vi "FPGAmacro6_2.vi"() -> ()   [LabVIEW 2019]
uses:
  <vilib>/Platform/TimedLoop/XDataNode/timing_clust.ctl
  <vilib>/Platform/TimedLoop/XDataNode/nitl_modes.ctl
  <vilib>/Platform/TimedLoop/XDataNode/wakeup.ctl
  <vilib>/rvi/Emulation/niFpgaGetClockAttributes.vi
  <vilib>/rvi/Emulation/niFpgaSctlEmulationGetInTimedLoop.vi
  <vilib>/rvi/Emulation/niFpgaEmulationReportErrorSimple.vi
  <vilib>/rvi/Emulation/niFpgaProcessEmulError.vi
  <vilib>/rvi/eio/common/nirviEmuTemplateMethod_errors.vi
  <vilib>/rvi/Emulation/niFpgaCriticalErrorInLSC.vi
  <vilib>/rvi/Memory/Memory_Emulation/nirvimemoryEmulation.vi
  <vilib>/rvi/Memory/Memory_Emulation/nirvimemoryFastEmulation.vi
  <vilib>/rvi/DataTransferAndStorage/Container/Common/niFpgaContainerGetUniqueNameForEmu.vi
  <vilib>/rvi/Memory/Memory_Emulation/niFpgaMemoryEmulationCacheClearOnFirstRun.vi
  <vilib>/rvi/Memory/Memory_Emulation/nirvimemoryEmulationManagerCache_MakeExclusive.vi
  <vilib>/rvi/Memory/Memory_Emulation/niFpgaMemoryEmulationValidateCache.vi
  <vilib>/rvi/Memory/Memory_Emulation/nirvimemoryEmulationManagerCache_InsertValue.vi
  <vilib>/Utility/error.llb/Clear Errors.vi
  <vilib>/rvi/Memory/Memory_Emulation/nirvimemoryEmulationManagerCache_ReleaseExclusive.vi
  <vilib>/rvi/Memory/Memory_Emulation/nirvimemoryEmulationManagerCache_GetValue.vi
  <vilib>/rvi/Emulation/niFpgaEmulationIsFPGAContextNoSignature.vi
  <vilib>/rvi/Memory/Memory_Emulation/nirvimemoryEmulationManagerCache_SetValue.vi
  <vilib>/rvi/Emulation/niFpgaSctlEmulationResourceMgr.vi
  <vilib>/rvi/DataTransferAndStorage/Container/Common/niFpgaContainerExecOnDevCompGetState.vi
  <vilib>/rvi/errors/niFpgaSetErrorForExecOnDevCompSimple.vi
  <vilib>/rvi/eio/common/nirviEmuReportErrorAndStop.vi
  <vilib>/rvi/FIFO/Fifo_Resource/nirvififoEmulationSetSize.vi
  <vilib>/rvi/FIFO/Fifo_Resource/nirviFifoEmulationQueueMgr.vi
  <instcachedir>/0/nirviFifoEmulationQueueMgr_E5CAEC123FF24DC58D834DCA3CDAA9B5.lvgen/nirviFifoEmulationQueueMgr_E5CAEC123FF24DC58D834DCA3CDAA9B5_001.vi
  <vilib>/rvi/FIFO/Fifo_Resource/nirvififoEmulationDetermineInputValidOut.vi
  <vilib>/rvi/FIFO/Fifo_Resource/nirvififoEmulationCreateLock.vi
  <vilib>/rvi/FIFO/Fifo_Resource/nirvififoEmulationObtainLock.vi
  <vilib>/rvi/FIFO/Fifo_Resource/nirvififoEmulationReleaseLock.vi
  <vilib>/rvi/occurrence/nirviWaitOnOccurrenceBase.vi
  <vilib>/rvi/errors/nirviReportUnexpectedCaseInternalError.vi
  <vilib>/rvi/errors/nirviReportUnexpectedCaseInternalError (U32).vi
  <vilib>/rvi/interface/RandomDataEmulation/niFpgaRandomDataHandleErrors.vi
  <vilib>/rvi/DataTransferAndStorage/Container/Common/niFpgaContainerSetEmuInfo.vi
  <vilib>/eio/EIONode/EIONode.xnode
  <vilib>/Platform/TimedLoop/XDataNode/XDataNode.xnode
  <vilib>/rvi/DataTransferAndStorage/Container/XNode/niFpgaContainer.xnode
  <vilib>/rvi/FIFO/Fifo_Resource/niFpgaFifoEmulationRefIn.vi
  <vilib>/rvi/interface/RandomDataEmulation/nirviRandomDataFpgaReadWriteTemplate.vi
  <vilib>/addons/control/pid/fpga.llb/XNode/niFpgaPID.xnode
  <vilib>/rvi/Analysis/common/FxpNativeNode/niFpgaFxpNative.xnode
  <vilib>/rvi/LocalResourceManager/LocalResourceManager.xnode
  <vilib>/Platform/TimedLoop/XDataNode/XDNodeRunTimeDep.lvlib
panel:
  in  "AO4 max":i16 min=0 max=3277
  in  "AO7":i16
  in  "AO6":i16
  in  "AO5":i16
  in  "Servo 3":bool
  in  "Servo 3 times":T1
  in  "Servo 2":bool
  in  "Servo 2 times":T1
  in  "Servo 1":bool
  in  "Servo 1 times":T1
  in  "Servo 0 times":T1
  in  "Servo 0":bool
  in  "Integral const":fxp<+/-,33,17> format="%.22g"
  out "Integrator input":fxp<+/-,48,32> format="%.26g"
  out "output":fxp<+/-,64,48> format="%.31g"
  in  "reset lock":bool
  in  "Setpoint":i16
  in  "Lock?":bool
  in  "Unlocked output":fxp<+/-,64,48> format="%.31g"
  in  "D31":bool
  in  "D30":bool
  in  "D29":bool
  in  "D28":bool
  in  "D27":bool
  in  "D26":bool
  in  "D25":bool
  in  "D24":bool
  out "Seq DO bits":u64
  in  "High power":bool
  in  "Reinitialise controller":bool
  in  "PID gains":T2={"Proportional gain Kc"=0.0, "Integral time Ti [min]"=2.0, "Derivative time Td [min]"=0.0}
  in  "Controller output range":T3={"Output high"=10.0, "Output low"=-10.0}
  out "Control Signal 2":i16
  in  "Setpoint (L)":fxp<+/-,16,16> format="%.3f"
  out "Filtered Input":fxp<+/-,16,16>
  out "Filtered Input":i16(graph)
  out "Control Signal":i16(graph)
  out "Input Signal / mV":fxp<+/-,19,14> format="%.3g"
  out "Control Signal / mV":fxp<+/-,19,14> format="%.3g"
  in  "Setpoint (H)":fxp<+/-,16,16>
  in  "override noise eater?":bool
  in  "D23":bool
  in  "D22":bool
  in  "D21":bool
  in  "D20":bool
  in  "D19":bool
  in  "D18":bool
  in  "D17":bool
  in  "D16":bool
  in  "D15":bool
  in  "D14":bool
  in  "D13":bool
  in  "D12":bool
  out "coerced AO3 fl scan":i16
  in  "AO3 fl scan":i16
  out "Seq AO bits":u8
  in  "trigger data":u8
  in  "AO data":u8
  in  "time data":u32
  in  "count data":u8
  out "data waiting":bool
  in  "pulse number":u32
  in  "digout data":u64
  in  "Send photons?":bool
  out "Numeric":u32
  out "Array":u32[](array[numeric])
  in  "DIO11":bool
  in  "DIO5":bool
  in  "DIO4":bool
  in  "dds/ag":bool
  in  "AO1":bool
  in  "AO1 off":i16
  in  "AO1 on":i16
  in  "AO4":bool
  in  "AO4 off":i16
  in  "AO4 on":i16
  out "PMT COUNTS D":u32
  out "PMT COUNTS C":u32
  in  "AO3":bool
  in  "AO2":bool
  in  "AO3 off":i16
  in  "AO2 off":i16
  in  "AO3 on":i16
  in  "AO2 on":i16
  out "Error type":u8
  out "Error?":bool
  in  "Fl scan time":u32
  in  "Enum":enum16{"Pulse", "Fluorescence"}(ring)
  out "bin number":u32
  in  "ticks per bin":u32=40000000
  out "Frequency Chart":u32(graph)
  out "loop counter":u64
  in  "AOM":bool
  in  "DIO10":bool
  in  "Microwave":bool
  in  "EOM":bool
  in  "DIO6":bool
  in  "DIO7":bool
  in  "DIO9":bool
  in  "DIO8":bool
  out "PMT saturation":bool
  out "Slave loop selector":u8
  in  "AO7":i16
  in  "AO6":i16
  in  "start sequence":bool
  in  "Line trig?":bool
  in  "# of pulses":i32
  in  "Debug counts?":bool
  in  "# of runs":i32
  out "Fifo Timed Out (B)":bool
  out "PMT COUNTS A":u32
  out "Fifo Timed Out (A)":bool
  out "PMT COUNTS B":u32
  # "Seb AO"
  # "Scan type:"
  # "Load AO memory"
  # "Fluorescence scan"
  # "Pulse sequencer"
  # "Globals"
  # "369 drift lock"
  # "List of error types:\n\n1: AO3 (AOM) voltage out of range."
  # "Crud:"
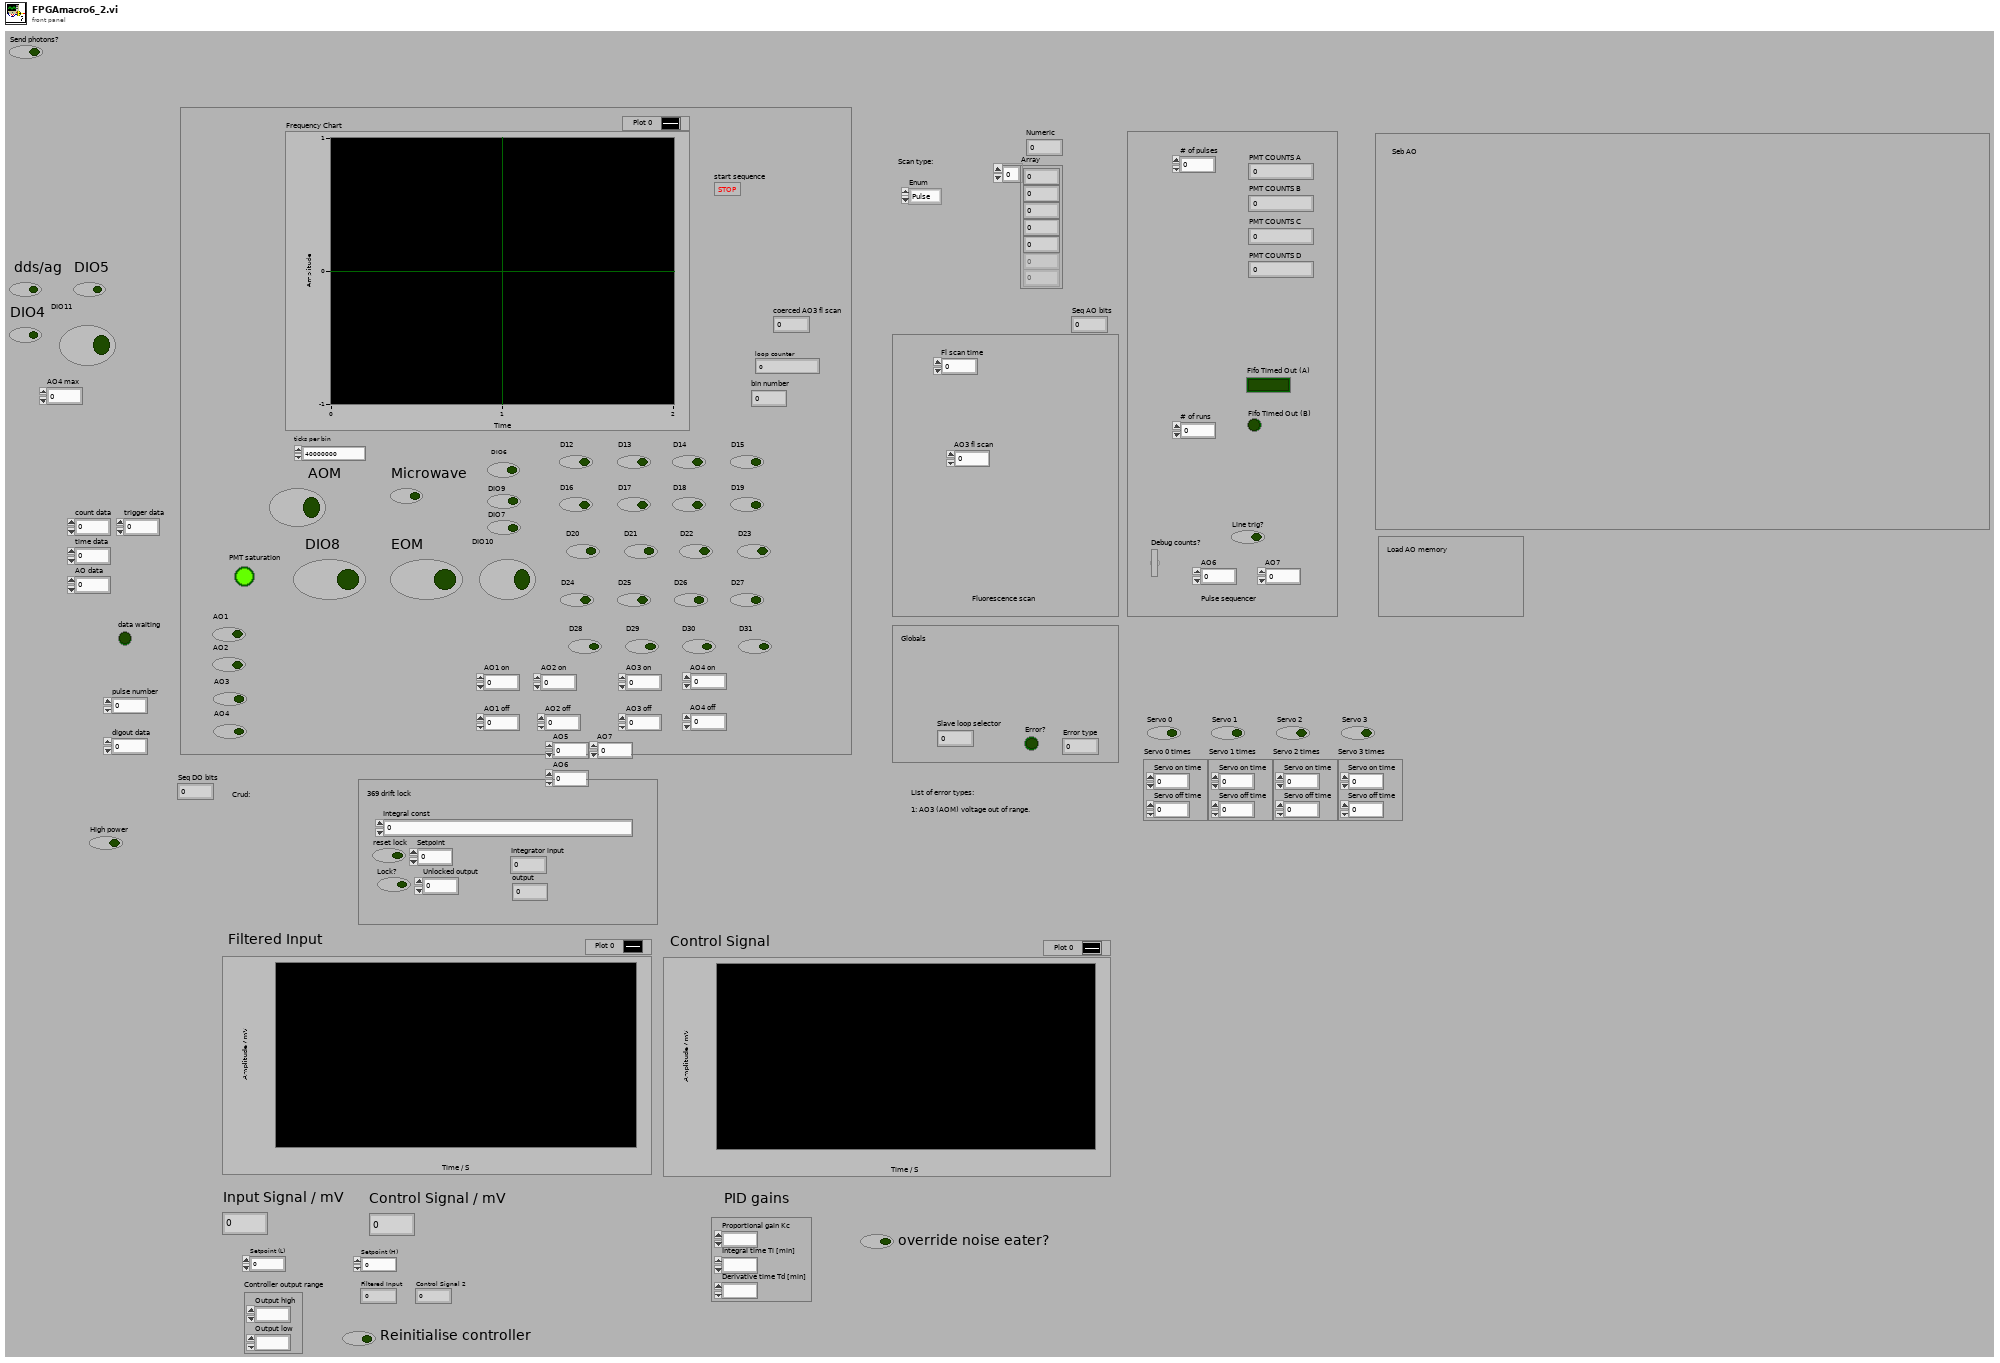
[diagram p1: front panel]
types:
  T1 = cluster{"Servo on time":u32, "Servo off time":u32}
  T2 = cluster{"Proportional gain Kc":fxp<+/-,16,8>, "Integral time Ti [min]":fxp<+/-,16,8>, "Derivative time Td [min]":fxp<+/-,16,8>}
  T3 = cluster{"Output high":fxp<+/-,16,16>, "Output low":fxp<+/-,16,16>}
  T4 = typedef "XDNodeRunTimeDep.lvlib/timing_clust.ctl" = cluster{"Expected End [f-1]":u64, "Actual End [f-1]":u64, "Finished Late? [f-1]":bool, "Expected End [i-1]":u64, "Actual End [i-1]":u64, "Finished Late? [i-1]":bool, "Expected Start [i]":u64, "Actual Start [i]":u64, "Expected Start [f]":u64, "Actual Start [f]":u64, "Source Name":string, "Structure Name":string, "Period":i64, "Deadline":i64, "Offset":i64, "Start":i64, "Priority":i32, "Timeout":i32, "Mode":T5, "Wakeup Reason":T6, "Error":errorcluster, "Source Type":string, "Secondary Source Type":string, "Global End Time":u64, "Global Start Time":u64, "Frame Duration":u64, "Iteration Duration":u64, "Assigned CPU":i32, "I/O Scan Engine Mode":u32}
  T5 = typedef "XDNodeRunTimeDep.lvlib/nitl_modes.ctl" = enum32{"No Change", "Process missed periods, maintain original phase", "Discard missed periods, maintain original phase", "Process missed periods, ignore original phase", "Discard missed periods, ignore original phase"}
  T6 = typedef "XDNodeRunTimeDep.lvlib/wakeup.ctl" = enum32{"Normal", "Aborted", "Asynchronous wakeup", "Timing source error", "Timed loop error", "Timeout"}
  T7 = cluster{"Boolean array[0]":bool, "Boolean array[1]":bool, "Boolean array[2]":bool, "Boolean array[3]":bool}
  T8 = cluster{"proportional gain (Kc)":i16, "integral gain (Kc*Ts/Ti)":i16, "derivative gain (Kc*Td/Ts)":i16}
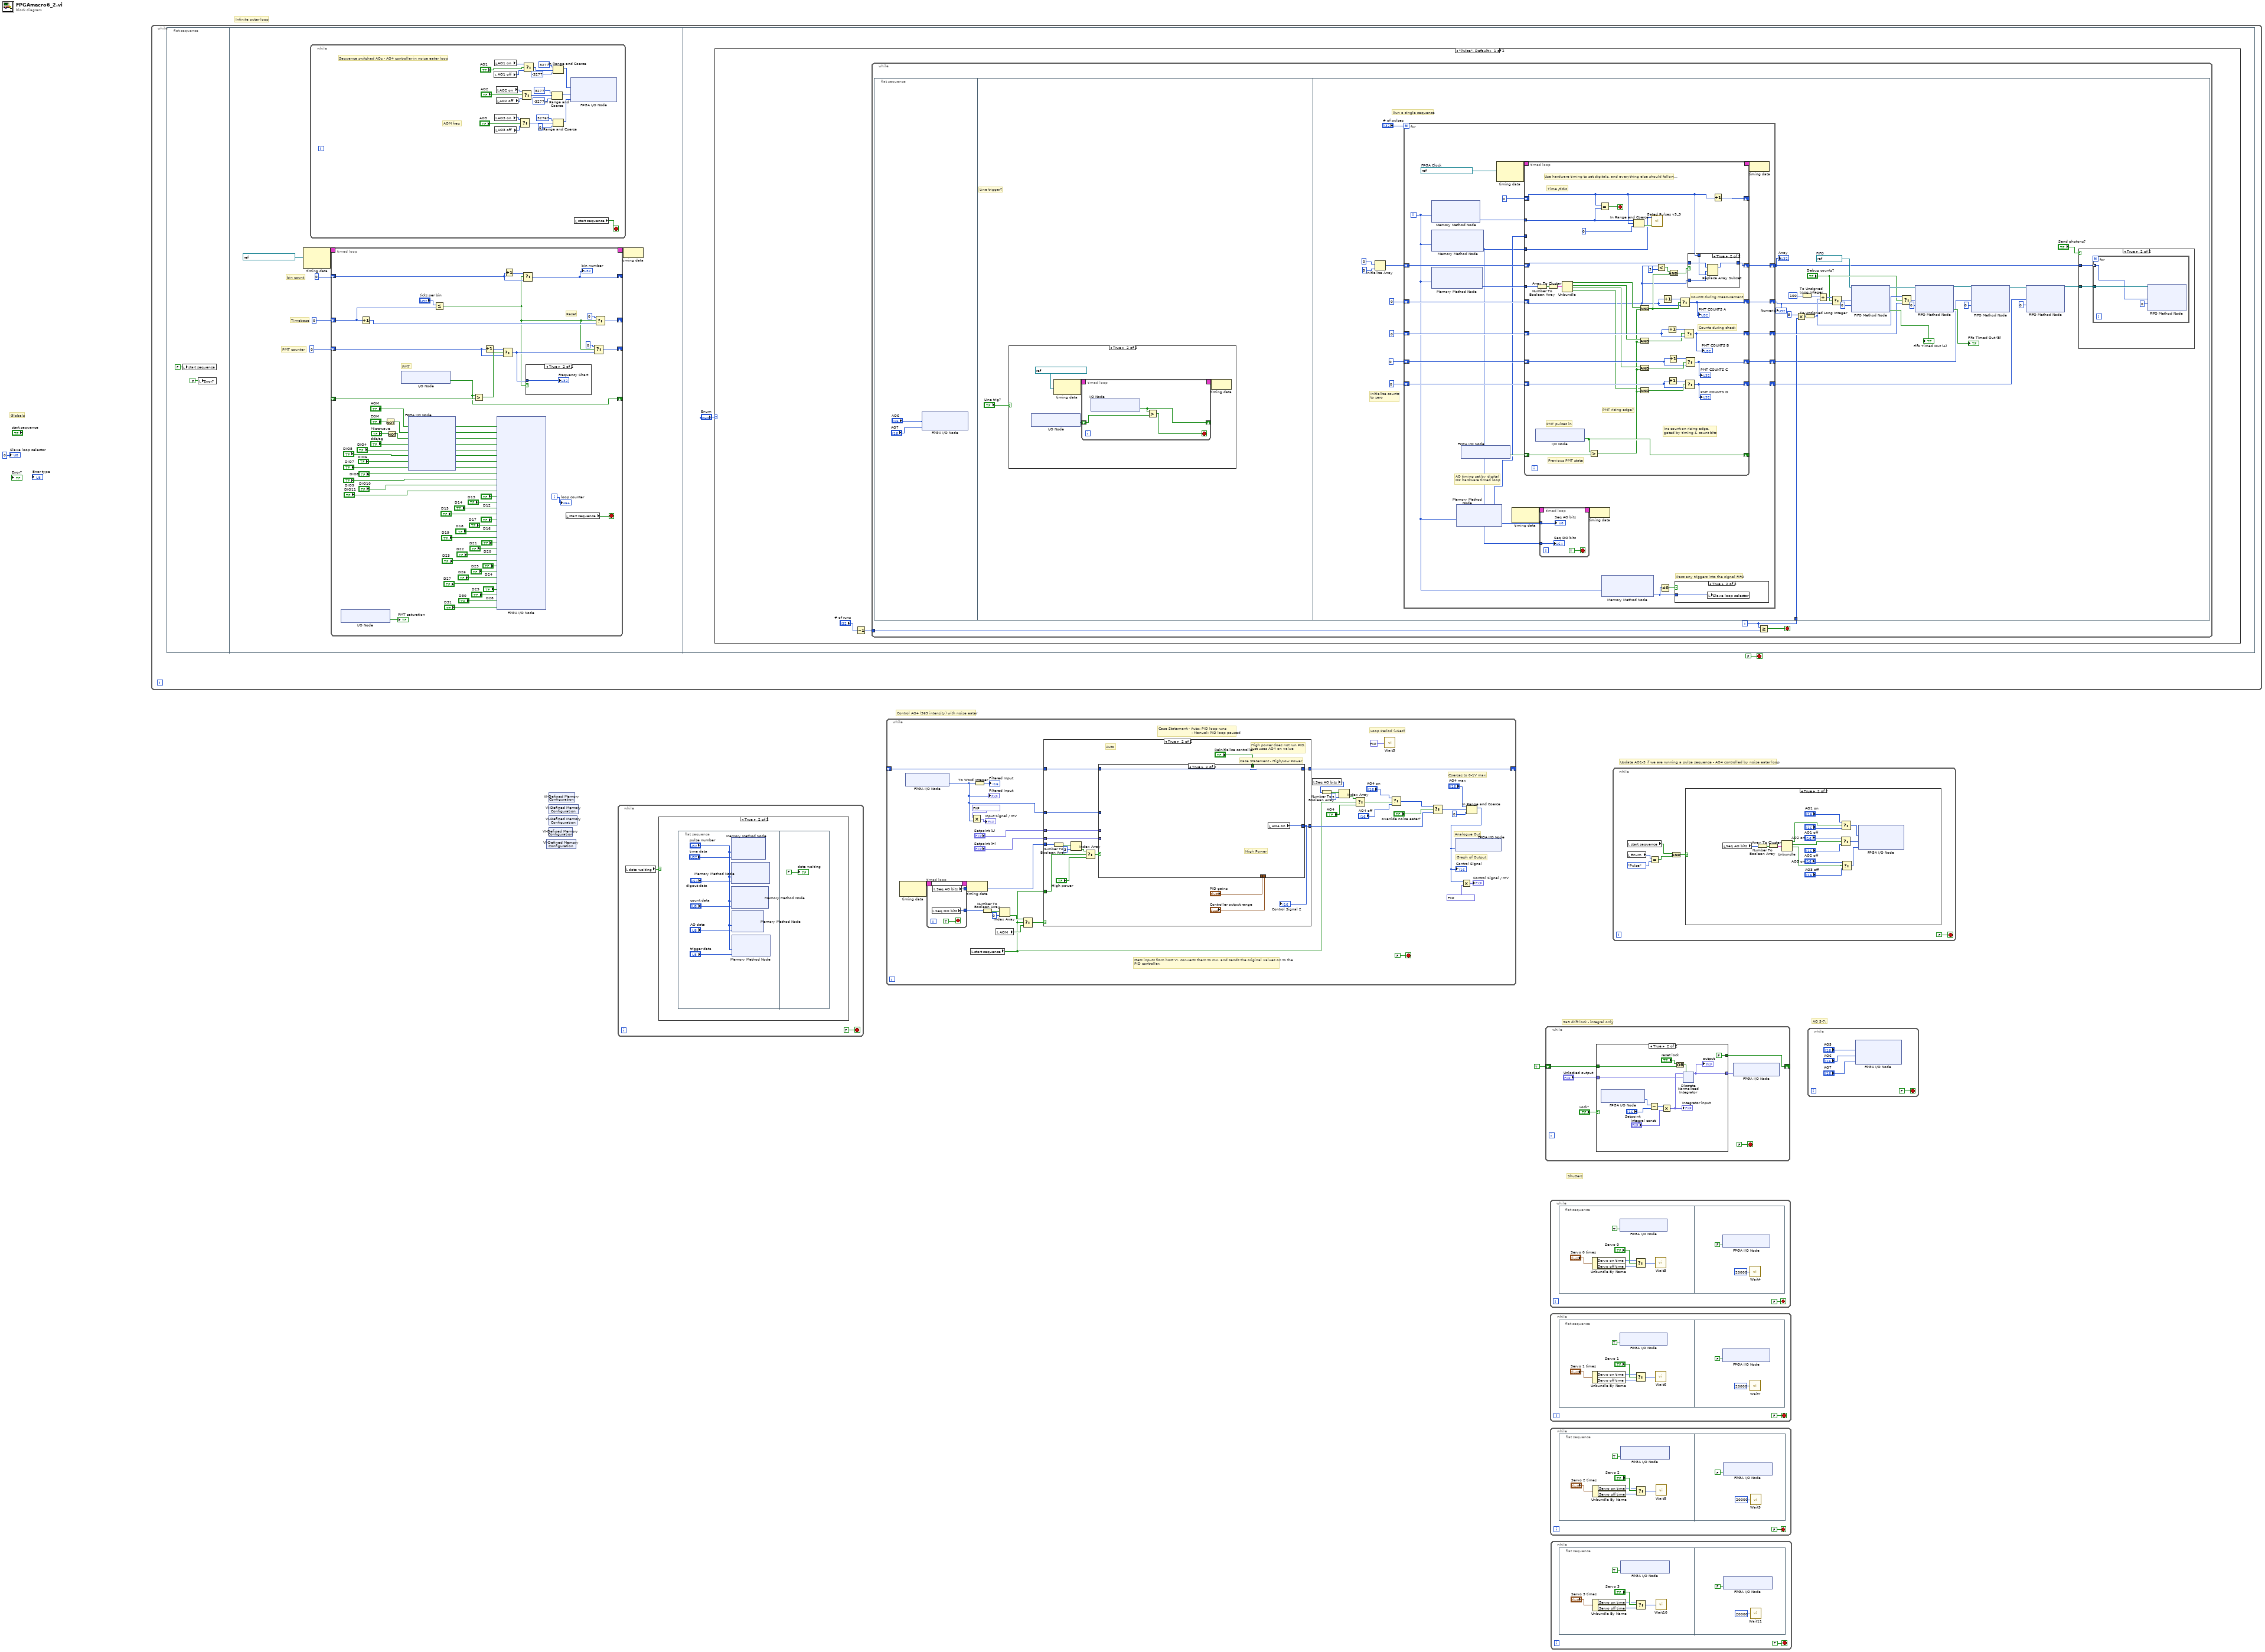
[diagram p0: block diagram]
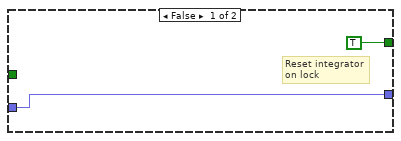
[diagram p2: hidden frame]
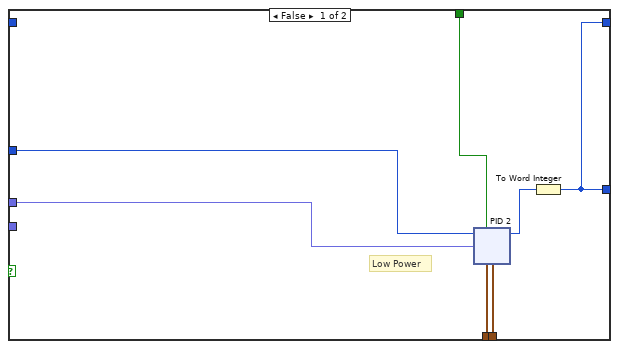
[diagram p4: hidden frame]
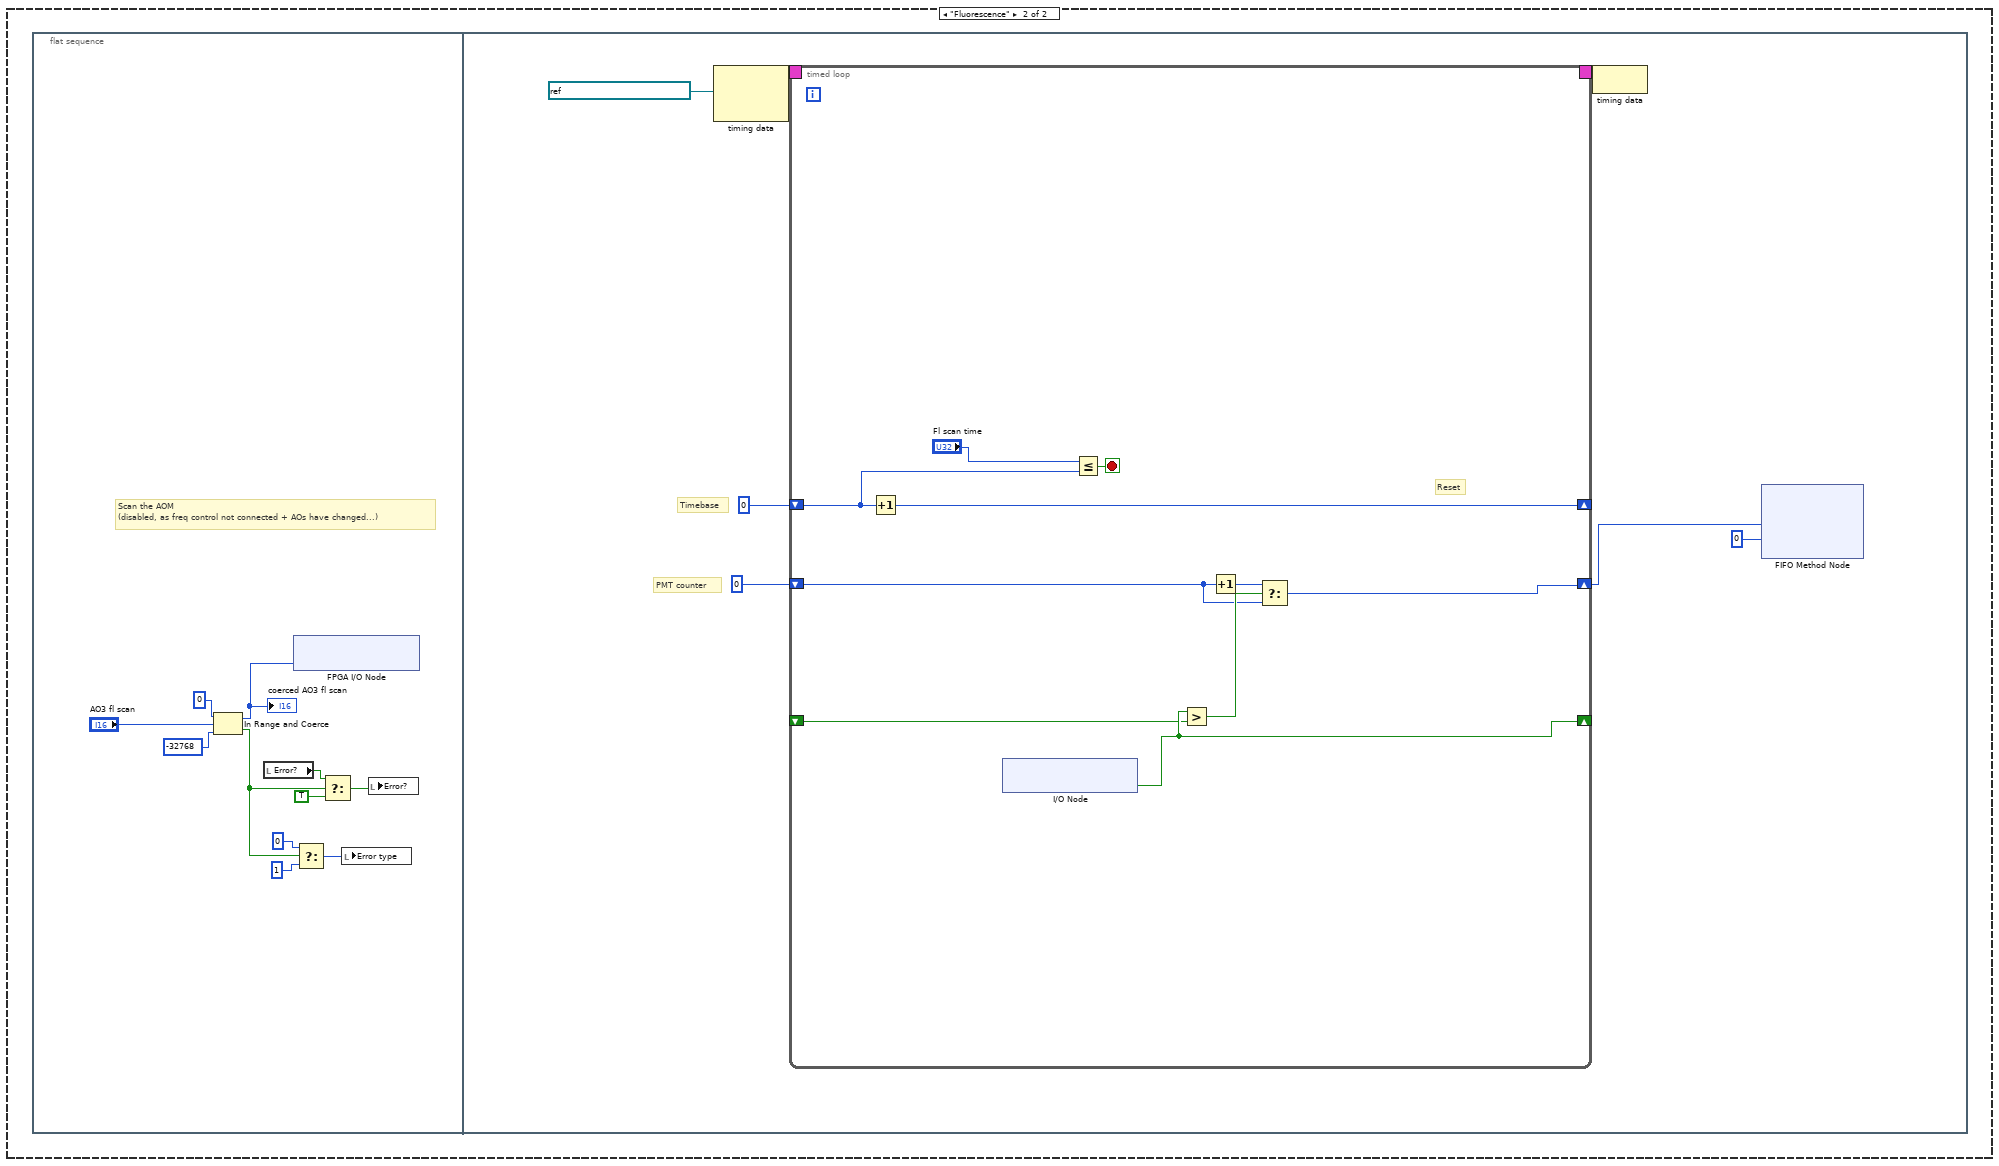
[diagram p12: hidden frame]
diagram:
  # "Control AO4 (369 intensity) with noise eater"
  # "Update AO1-3 if we are running a pulse sequence - AO4 controlled by noise eater loop"
  # "AO 5-7:"
  # "Shutters"
  # "369 drift lock - integral only"
  # "Globals"
  # "Infinite outer loop"
  n1 = while {
    stop <- FALSE stop-if-true
    n2 = flat-sequence {
      frame #0 {
        n3 = local write "start sequence"(FALSE ("start sequence")) -> ()
        n4 = local write "Error?"(FALSE ("Error?")) -> ()
      }
      frame #1 {
        # "bin count"
        # "PMT counter"
        # "Timebase"
        n5 = node-c288(refnum<k21> "40 MHz Onboard Clock" ("FPGA Clock To Enable")) -> (w11:T4)  [unwired: 1 in]
        n6 = while {
          stop <- w94 stop-if-true
          # "AOM freq"
          # "Sequence switched AOs - AO4 controller in noise eater loop"
          n7 = local read "AO1 off"() -> (w76:i16)
          n8 = local read "AO1 on"() -> (w77:i16)
          n9 = local read "AO3 on"() -> (w87:i16)
          n10 = local read "AO3 off"() -> (w86:i16)
          n11 = local read "AO2 on"() -> (w89:i16)
          n12 = local read "AO2 off"() -> (w88:i16)
          n13 = Select(t=w87, s="AO3", f=w86) -> (s? t:f=w83:i16)
          n14 = Select(t=w89, s="AO2", f=w88) -> (s? t:f=w82:i16)
          n15 = Select(t=w77, s="AO1", f=w76) -> (s? t:f=w78:i16)
          n16 = In Range and Coerce(upper limit=i16 3277, x=w82, lower limit=i16 -3277) -> (coerced(x)=w93:i16)  [unwired: 1 out]
          n17 = In Range and Coerce(upper limit=i16 32767, x=w83, lower limit=i16 0) -> (coerced(x)=w90:i16)  [unwired: 1 out]
          n18 = In Range and Coerce(upper limit=i16 3277, x=w78, lower limit=i16 -3277) -> (coerced(x)=w79:i16)  [unwired: 1 out]
          n19 = xnode "FPGA I/O Node"("Connector0/AO1"=w79, "Connector0/AO2"=w93, "Connector0/AO3"=w90) -> ()  [unwired: 3 in, 3 out]
          n20 = local read "start sequence"() -> (w94:bool)
        }
        n21 = timed-loop {
          timing: w11 -> [_]
          timing-out: [_] -> w10
          shift-right: [w63] -> _
          shift-left: u32 0 -> [w56]
          shift-right: [w61] -> _
          shift-left: u32 0 -> [w58]
          shift-right: [w46] -> _
          shift-left: _ -> [w54]
          shift-right: [w50] -> _
          shift-left: u32 0 -> [w48]
          i -> [w55]
          stop <- w51 stop-if-true
          # "PMT"
          # "Reset"
          n22 = xnode "I/O Node"() -> ("Connector0/DIO13"=→"PMT saturation":bool)  [unwired: 1 in, 1 out]
          n23 = Increment(x=w56) -> (x+1=w65:u32)
          n24 = Not(x="EOM") -> (.not. x?=w13:bool)
          n25 = Not(x="Microwave") -> (.not. x?=w44:bool)
          n26 = xnode "I/O Node"() -> ("Connector0/DIO15"=w46:bool)  [unwired: 1 in, 1 out]
          n27 = xnode "FPGA I/O Node"("Connector0/DIO0"="AOM", "Connector0/DIO1"=w13, "Connector0/DIO2"=w44, "Connector0/DIO3"="dds/ag", "Connector0/DIO4"="DIO4", "Connector0/DIO5"="DIO5", "Connector0/DIO6"="DIO6", "Connector0/DIO7"="DIO7") -> ()  [unwired: 8 in, 8 out]
          n28 = Less Or Equal?(x="ticks per bin", y=w56) -> (x <= y?=w47:bool)
          n29 = Greater?(x=w46, y=w54) -> (0:w59:bool)
          n30 = Increment(x=w58) -> (x+1=w62:u32)
          n31 = xnode "FPGA I/O Node"("Connector1/DIO0"="AOM", "Connector1/DIO1"=w13, "Connector1/DIO2"=w44, "Connector1/DIO3"="dds/ag", "Connector1/DIO4"="DIO4", "Connector1/DIO5"="DIO5", "Connector1/DIO6"="DIO6", "Connector1/DIO7"="DIO7", "Connector1/DIO8"="DIO8", "Connector1/DIO9"="DIO9", "Connector1/DIO10"="DIO10", "Connector1/DIO11"="DIO11", "Connector1/DIO12"="D12", "Connector1/DIO13"="D13", "Connector1/DIO14"="D14", "Connector1/DIO15"="D15", "Connector1/DIO16"="D16", "Connector1/DIO17"="D17", "Connector1/DIO18"="D18", "Connector1/DIO19"="D19", "Connector1/DIO20"="D20", "Connector1/DIO21"="D21", "Connector1/DIO22"="D22", "Connector1/DIO23"="D23", "Connector1/DIO24"="D24", "Connector1/DIO25"="D25", "Connector1/DIO26"="D26", "Connector1/DIO27"="D27", "Connector1/DIO28"="D28", "Connector1/DIO29"="D29", "Connector1/DIO30"="D30", "Connector1/DIO31"="D31") -> ()  [unwired: 32 in, 32 out]
          n32 = Select(t=w62, s=w59, f=w58) -> (s? t:f=w52:u32)
          n33 = Increment(x=w48) -> (x+1=w49:u32)
          n34 = Select(t=w49, s=w47, f=w48) -> (s? t:f=w50:u32)
          "bin number" <- w50
          n35 = case shown="True" w47 {
            tunnel: w52 -> [_ w66]
            frame False {
            }
            frame True {
              "Frequency Chart" <- w66
            }
          }
          n36 = local read "start sequence"() -> (w51:bool)
          n37 = Select(t=u32 0, s=w47, f=w52) -> (s? t:f=w61:u32)
          n38 = Select(t=u32 0, s=w47, f=w65) -> (s? t:f=w63:u32)
          "loop counter" <- w55
        }
        n39 = node-c288(w10) -> ()
      }
      frame #2 {
        n40 = case shown="\"Pulse\", Default" "Enum" {
          frame "Pulse", Default {
            n41 = Decrement(x="# of runs") -> (x-1=w96:i32)
            n42 = while {
              tunnel: w96 -> [w99]
              i -> [w100]
              stop <- w98 stop-if-true
              n43 = flat-sequence {
                tunnel: w100 -> [w132]
                frame #0 {
                  n44 = xnode "FPGA I/O Node"("Connector0/AO6"="AO6", "Connector0/AO7"="AO7") -> ()  [unwired: 2 in, 2 out]
                }
                frame #1 {
                  # "Line trigger?"
                  n45 = case shown="True" "Line trig?" {
                    frame False {
                    }
                    frame True {
                      n46 = xnode "I/O Node"() -> ("Connector0/DIO14"=w104:bool)  [unwired: 1 in, 1 out]
                      n47 = node-c288(refnum<k21> "40 MHz Onboard Clock" ("Source Name")) -> (w107:T4)
                      n48 = timed-loop {
                        timing: w107 -> [_]
                        timing-out: [_] -> w106
                        shift-right: [w109] -> _
                        shift-left: w104 -> [w110]
                        stop <- w108 stop-if-true
                        n49 = xnode "I/O Node"() -> ("Connector0/DIO14"=w109:bool)  [unwired: 1 in, 1 out]
                        n50 = Greater?(x=w109, y=w110) -> (0:w108:bool)
                      }
                      n51 = node-c288(w106) -> ()
                    }
                  }
                }
                frame #2 {
                  w120 = refnum<k21> "U32 FIFO"  # FIFO
                  # "Run a single sequence"
                  # "Initialize counts\nto zero"
                  n52 = Initialize Array(u32 0 ("element"), 5 ("dimension size")) -> (w121:u32[])
                  n53 = for {
                    N: "# of pulses" -> [_]
                    shift-right: [w177] -> w138
                    shift-left: u32 0 -> [w175]
                    shift-right: [w176] -> w140
                    shift-left: u32 0 -> [w174]
                    shift-right: [w169] -> w125
                    shift-left: u32 0 -> [w170]
                    shift-right: [w167] -> w124
                    shift-left: u32 0 -> [w168]
                    shift-right: [w165] -> w117
                    shift-left: w121 -> [w166]
                    i -> [w162]
                    w178 = refnum<k21> "40 MHz Onboard Clock"  # FPGA Clock
                    # "AO timing set by digital\nOP hardware timed loop"
                    # "Pass any triggers into the signal FIFO"
                    n54 = xnode ("Memory Method Node")("Address"=w162) -> ("Data"=w159:u64)  [unwired: 1 in, 1 out]
                    n55 = xnode ("Memory Method Node")("Address"=w162) -> ("Data"=w164:u32)  [unwired: 1 in, 1 out]
                    n56 = xnode ("Memory Method Node")("Address"=w162) -> ("Data"=w163:u8)  [unwired: 1 in, 1 out]
                    n57 = xnode ("Memory Method Node")("Address"=w162) -> ("Data"=w161:u8)  [unwired: 1 in, 1 out]
                    n58 = xnode "FPGA I/O Node"() -> ("Connector0/DIO15"=w172:bool)  [unwired: 1 in, 1 out]
                    n59 = node-c288(w178) -> (w180:T4)  [unwired: 1 in]
                    n60 = node-c288() -> (w158:T4)  [unwired: 1 in]
                    n61 = timed-loop {
                      timing: w180 -> [_]
                      timing-out: [_] -> w179
                      shift-right: [w220] -> w177
                      shift-left: w175 -> [w190]
                      shift-right: [w226] -> _
                      shift-left: w172 -> [w225]
                      shift-right: [w210] -> _
                      shift-left: u32 0 -> [w189]
                      shift-right: [w218] -> w176
                      shift-left: w174 -> [w222]
                      tunnel: w159 -> [w212]
                      tunnel: w163 -> [w211]
                      tunnel: w164 -> [w209]
                      shift-right: [w203] -> w169
                      shift-left: w170 -> [w205]
                      shift-right: [w199] -> w167
                      shift-left: w168 -> [w200]
                      shift-right: [w191] -> w165
                      shift-left: w166 -> [w193]
                      tunnel: w161 -> [_]
                      stop <- w219 stop-if-true
                      # "Use hardware timing to set digitals, and everything else should follow..."
                      # "Previous PMT state"
                      # "Counts during check"
                      # "Counts during measurement"
                      # "Time /ticks"
                      # "Inc count on rising edge,\ngated by timing & count bits"
                      # "PMT rising edge?"
                      # "PMT pulses in"
                      n62 = xnode "I/O Node"() -> ("Connector0/DIO15"=w226:bool)  [unwired: 1 in, 1 out]
                      n63 = Number To Boolean Array(number=w211) -> (Boolean array=w215:bool[])
                      n64 = Array To Cluster(array=w215) -> (cluster=w214:T7)
                      n65 = Unbundle(w214) -> ("Boolean array[0]"=w208:bool, "Boolean array[1]"=w213:bool, "Boolean array[2]"=w204:bool, "Boolean array[3]"=w197:bool)
                      n66 = Greater?(x=w226, y=w225) -> (0:w198:bool)
                      n67 = Equal?(x=w189, y=w209) -> (x = y?=w219:bool)
                      n68 = In Range and Coerce(upper limit=w209, x=w189, lower limit=u32 0) -> (In Range?=w217:bool)  [unwired: 1 out]
                      n69 = And(x=w208, y=w198) -> (x .and. y?=w194:bool)
                      n70 = And(x=w213, y=w198) -> (x .and. y?=w221:bool)
                      n71 = And(x=w204, y=w198) -> (x .and. y?=w206:bool)
                      n72 = And(x=w197, y=w198) -> (x .and. y?=w201:bool)
                      n73 = call "Gated Pulses v5_9.vi"("Gate"=w217, "Pulse bits"=w212) -> ()  [unwired: 3 in]
                      n74 = Less?(x=w190, y=i16 5) -> (x < y?=w195:bool)
                      n75 = Increment(x=w190) -> (x+1=w224:u32)
                      n76 = Increment(x=w222) -> (x+1=w223:u32)
                      n77 = Increment(x=w200) -> (x+1=w202:u32)
                      n78 = Increment(x=w205) -> (x+1=w207:u32)
                      n79 = And(x=w195, y=w194) -> (x .and. y?=w192:bool)
                      n80 = Select(t=w224, s=w194, f=w190) -> (s? t:f=w220:u32)
                      "PMT COUNTS A" <- w220
                      n81 = Select(t=w223, s=w221, f=w222) -> (s? t:f=w218:u32)
                      "PMT COUNTS B" <- w218
                      n82 = Select(t=w202, s=w201, f=w200) -> (s? t:f=w199:u32)
                      "PMT COUNTS D" <- w199
                      n83 = Select(t=w207, s=w206, f=w205) -> (s? t:f=w203:u32)
                      "PMT COUNTS C" <- w203
                      n84 = case shown="True" w192 {
                        tunnel: w193 -> [w227 w231]
                        tunnel: [w227 w230] -> w191
                        tunnel: w190 -> [_ w228]
                        tunnel: w189 -> [_ w229]
                        frame False {
                        }
                        frame True {
                          n85 = Replace Array Subset(array=w231, new element=w229, index=w228) -> (w230:u32[])
                        }
                      }
                      n86 = Increment(x=w189) -> (x+1=w210:u32)
                    }
                    n87 = timed-loop {
                      timing: w158 -> [_]
                      timing-out: [_] -> w157
                      tunnel: w161 -> [w183]
                      tunnel: w159 -> [w182]
                      stop <- TRUE stop-if-true
                      "Seq AO bits" <- w183
                      "Seq DO bits" <- w182
                    }
                    n88 = node-c288(w157) -> ()
                    n89 = xnode ("Memory Method Node")("Address"=w162) -> ("Data"=w160:u8)  [unwired: 1 in, 1 out]
                    n90 = Not Equal To 0?(x=w160) -> (x != 0?=w171:bool)
                    n91 = case shown="True" w171 {
                      tunnel: w160 -> [_ w188]
                      frame False {
                      }
                      frame True {
                        n92 = local write "Slave loop selector"(w188) -> ()
                      }
                    }
                    n93 = node-c288(w179) -> ()
                  }
                  "Array" <- w117
                  "Numeric" <- w138
                  n94 = Multiply(x=5 ("y"), y=w132) -> (x*y=w145:i32)
                  n95 = To Unsigned Long Integer(number=i16 100) -> (unsigned 32bit integer=w146:u32)
                  n96 = To Unsigned Long Integer(number=w145) -> (unsigned 32bit integer=w144:u32)
                  n97 = Add(x=w146, y=w144) -> (x+y=w142:u32)
                  n98 = Select(t=w142, s="Debug counts?", f=w138) -> (s? t:f=w141:u32)
                  n99 = xnode ("FIFO Method Node")("Element"=w141, "Timeout"=0, "FIFO In"=w120) -> ("Timed Out?"=→"Fifo Timed Out (A)":bool, "FIFO Out"=w149:refnum<k21>)
                  n100 = Select(t=w144, s="Debug counts?", f=w140) -> (s? t:f=w143:u32)
                  n101 = xnode ("FIFO Method Node")("Element"=w143, "Timeout"=0, "FIFO In"=w149) -> ("Timed Out?"=→"Fifo Timed Out (B)":bool, "FIFO Out"=w129:refnum<k21>)
                  n102 = xnode ("FIFO Method Node")("Element"=w125, "Timeout"=0, "FIFO In"=w129) -> ("FIFO Out"=w128:refnum<k21>)  [unwired: 1 out]
                  n103 = xnode ("FIFO Method Node")("Element"=w124, "Timeout"=0, "FIFO In"=w128) -> ("FIFO Out"=w118:refnum<k21>)  [unwired: 1 out]
                  n104 = case shown="True" "Send photons?" {
                    tunnel: w118 -> [_ w153]
                    tunnel: w117 -> [_ w152]
                    frame False {
                    }
                    frame True {
                      n105 = for {
                        tunnel: w153 -> [w156]
                        tunnel: w152 -> [w154] mode=indexing
                        n106 = xnode ("FIFO Method Node")("Element"=w154, "Timeout"=0, "FIFO In"=w156) -> ()  [unwired: 2 out]
                      }
                    }
                  }
                }
              }
              n107 = Greater Or Equal?(x=w100, y=w99) -> (x >= y?=w98:bool)
            }
          }
          frame "Fluorescence" {
            n108 = flat-sequence {
              frame #0 {
                # "Scan the AOM\n(disabled, as freq control not connected + AOs have changed...)"
                n109 = In Range and Coerce(upper limit=i16 0, x="AO3 fl scan", lower limit=i16 -32768) -> (coerced(x)=w246:i16, In Range?=w241:bool)
                "coerced AO3 fl scan" <- w246
                n110 = local read "Error?"() -> (w245:bool)
                n111 = xnode "FPGA I/O Node"("Connector0/AO3"=w246) -> ()  [unwired: 1 in, 1 out]
                n112 = Select(t=u8 0, s=w241, f=u8 1) -> (s? t:f=w242:u8)
                n113 = Select(t=w245, s=w241, f=TRUE) -> (s? t:f=w243:bool)
                n114 = local write "Error type"(w242) -> ()
                n115 = local write "Error?"(w243) -> ()
              }
              frame #1 {
                # "PMT counter"
                # "Timebase"
                n116 = node-c288(refnum<k21> "40 MHz Onboard Clock" ("FPGA Clock To Enable")) -> (w255:T4)  [unwired: 1 in]
                n117 = timed-loop {
                  timing: w255 -> [_]
                  timing-out: [_] -> w254
                  shift-right: [w256] -> _
                  shift-left: u32 0 -> [w262]
                  shift-right: [w258] -> w249
                  shift-left: u32 0 -> [w263]
                  shift-right: [w261] -> _
                  shift-left: _ -> [w260]
                  stop <- w257 stop-if-true
                  # "Reset"
                  n118 = Increment(x=w262) -> (x+1=w256:u32)
                  n119 = xnode "I/O Node"() -> ("Connector0/DIO15"=w261:bool)  [unwired: 1 in, 1 out]
                  n120 = Less Or Equal?(x="Fl scan time", y=w262) -> (x <= y?=w257:bool)
                  n121 = Greater?(x=w261, y=w260) -> (0:w264:bool)
                  n122 = Increment(x=w263) -> (x+1=w265:u32)
                  n123 = Select(t=w265, s=w264, f=w263) -> (s? t:f=w258:u32)
                }
                n124 = node-c288(w254) -> ()
                n125 = xnode ("FIFO Method Node")("Element"=w249, "Timeout"=0) -> ()  [unwired: 1 in, 2 out]
              }
            }
          }
        }
      }
    }
  }
  n126 = xnode "VI-Defined Memory Configuration"() -> ()  [unwired: 1 out]
  n127 = xnode "VI-Defined Memory Configuration"() -> ()  [unwired: 1 out]
  n128 = xnode "VI-Defined Memory Configuration"() -> ()  [unwired: 1 out]
  n129 = xnode "VI-Defined Memory Configuration"() -> ()  [unwired: 1 out]
  n130 = xnode "VI-Defined Memory Configuration"() -> ()  [unwired: 1 out]
  n131 = while {
    stop <- FALSE stop-if-true
    n132 = local read "data waiting"() -> (w273:bool)
    n133 = case shown="True" w273 {
      frame False {
      }
      frame True {
        n134 = flat-sequence {
          frame #0 {
            n135 = xnode ("Memory Method Node")("Address"="pulse number", "Data"="time data") -> ()  [unwired: 1 in, 1 out]
            n136 = xnode ("Memory Method Node")("Address"="pulse number", "Data"="digout data") -> ()  [unwired: 1 in, 1 out]
            n137 = xnode ("Memory Method Node")("Address"="pulse number", "Data"="count data") -> ()  [unwired: 1 in, 1 out]
            n138 = xnode ("Memory Method Node")("Address"="pulse number", "Data"="AO data") -> ()  [unwired: 1 in, 1 out]
            n139 = xnode ("Memory Method Node")("Address"="pulse number", "Data"="trigger data") -> ()  [unwired: 1 in, 1 out]
          }
          frame #1 {
            "data waiting" <- FALSE
          }
        }
      }
    }
  }
  n140 = while {
    shift-right: [w293] -> _
    shift-left: _ -> [w292]
    stop <- FALSE stop-if-true
    # "Coerces to 0-1V max"
    # "Graph of Output"
    # "Gets inputs from host VI, converts them to mV, and sends the original values on to the PID controller."
    # "Case Statement - Auto: PID loop runs\n                            - Manual: PID loop paused"
    # "Analogue Out"
    # "Loop Period (uSec)"
    n141 = node-c288() -> (w295:T4)  [unwired: 1 in]
    n142 = xnode "FPGA I/O Node"() -> ("Connector0/AI0"=w281:i16)  [unwired: 1 in, 1 out]
    "Filtered Input" <- w281
    n143 = timed-loop {
      timing: w295 -> [_]
      timing-out: [_] -> w294
      tunnel: [w320] -> w307
      tunnel: [w319] -> w296
      stop <- TRUE stop-if-true
      n144 = local read "Seq DO bits"() -> (w320:u64)
      n145 = local read "Seq AO bits"() -> (w319:u8)
    }
    n146 = node-c288(w294) -> ()
    n147 = local read "start sequence"() -> (w297:bool)
    n148 = Multiply(x=fxp<+,10,-1> 0.30517578125, y=w281) -> (x*y=→"Input Signal / mV":fxp<+/-,26,15>)
    n149 = To Word Integer(number=w281) -> (16bit integer=→"Filtered Input":i16)
    n150 = Number To Boolean Array(number=w307) -> (Boolean array=w309:bool[])
    n151 = local read "AOM"() -> (w306:bool)
    n152 = Index Array(array=w309, index=0) -> (element=w304:bool)
    n153 = Select(t=w304, s=w297, f=w306) -> (s? t:f=w305:bool)
    n154 = case shown="True" w305 {
      tunnel: [w325 w330] -> w310
      tunnel: "Setpoint (L)" -> [_ w338]
      tunnel: "Setpoint (H)" -> [_ w337]
      tunnel: w297 -> [_ w336]
      tunnel: w296 -> [_ w329]
      tunnel: [w325 w328] -> w293
      tunnel: w292 -> [w325 w327]
      tunnel: w281 -> [_ w326]
      frame False {
        # "Manual"
      }
      frame True {
        # "High power does not run PID,\njust uses AO4 on value"
        # "Case Statement - High/Low Power"
        # "Auto"
        n155 = Number To Boolean Array(number=w329) -> (Boolean array=w332:bool[])
        n156 = Index Array(array=w332, index=3) -> (element=w331:bool)
        n157 = Select(t=w331, s=w336, f="High power") -> (s? t:f=w335:bool)
        n158 = case shown="True" w335 {
          tunnel: "Reinitialise controller" -> [w346 _]
          tunnel: "PID gains" -> [w348 _]
          tunnel: "Controller output range" -> [w347 _]
          tunnel: [w343 w378] -> w330
          tunnel: w338 -> [w345 _]
          tunnel: w337 -> [_ _]
          tunnel: [w343 w377] -> w328
          tunnel: w327 -> [_ w377]
          tunnel: w326 -> [w342 _]
          frame False {
            # "Low Power"
            n159 = xnode ("PID 2")("process variable"=w342, "reset?"=w346, "setpoint"=w345, "PID gains"=w348, "output range"=w347) -> ("output"=w344:i16)
            n160 = To Word Integer(number=w344) -> (16bit integer=w343:i16)
          }
          frame True {
            # "High Power"
            n161 = local read "AO4 on"() -> (w378:i16)
          }
        }
        "Control Signal 2" <- w330
      }
    }
    n162 = local read "Seq AO bits"() -> (w301:u8)
    n163 = Number To Boolean Array(number=w301) -> (Boolean array=w302:bool[])
    n164 = Index Array(array=w302, index=3) -> (element=w298:bool)
    n165 = Select(t=w298, s=w297, f="AO4") -> (s? t:f=w299:bool)
    n166 = call "Wait3"("Count(uSec)"=fxp<+,1,4> 8.0) -> ()  [unwired: 1 out]
    n167 = Select(t="AO4 on", s=w299, f="AO4 off") -> (s? t:f=w300:i16)
    n168 = Select(t=w300, s="override noise eater?", f=w310) -> (s? t:f=w288:i16)
    n169 = In Range and Coerce(upper limit="AO4 max", x=w288, lower limit=i16 0) -> (coerced(x)=w287:i16)  [unwired: 1 out]
    "Control Signal" <- w287
    n170 = xnode "FPGA I/O Node"("Connector0/AO4"=w287) -> ()  [unwired: 1 in, 1 out]
    n171 = Multiply(x=w287, y=fxp<+,10,-1> 0.30517578125) -> (x*y=→"Control Signal / mV":fxp<+/-,26,15>)
  }
  n172 = while {
    shift-right: [w381] -> _
    shift-left: TRUE -> [w380]
    stop <- FALSE stop-if-true
    n173 = case shown="True" "Lock?" {
      tunnel: [w386 w392] -> w379
      tunnel: "Unlocked output" -> [w386 w393]
      tunnel: [TRUE FALSE] -> w381
      tunnel: w380 -> [_ w389]
      frame False {
        # "Reset integrator\non lock"
      }
      frame True {
        n174 = xnode "FPGA I/O Node"() -> ("Connector0/AI1"=w387:i16)  [unwired: 1 in, 1 out]
        n175 = Subtract(x=w387, y="Setpoint") -> (x-y=w394:i16)
        n176 = Multiply(x=w394, y="Integral const") -> (x*y=w396:fxp<+/-,48,32>)
        "Integrator input" <- w396
        n177 = Or(x="reset lock", y=w389) -> (x .or. y?=w391:bool)
        n178 = xnode ("Discrete Normalized Integrator")("initial condition"=w393, "input"=w396, "reset"=w391) -> ("output"=w392:fxp<+/-,64,48>)
        "output" <- w392
      }
    }
    n179 = xnode "FPGA I/O Node"("Connector0/AO1"=w379) -> ()  [unwired: 1 in, 1 out]
  }
  n180 = while {
    stop <- FALSE stop-if-true
    n181 = flat-sequence {
      frame #0 {
        n182 = Unbundle By Name("Servo 0 times") -> ("Servo on time"=w414:u32, "Servo off time"=w413:u32)
        n183 = xnode "FPGA I/O Node"("Connector0/DIO8"=TRUE ("Connector1/DIO39")) -> ()  [unwired: 1 in, 1 out]
        n184 = Select(t=w414, s="Servo 0", f=w413) -> (s? t:f=w416:u32)
        n185 = call "Wait5"("Count(uSec)"=w416) -> ()  [unwired: 1 out]
      }
      frame #1 {
        n186 = xnode "FPGA I/O Node"("Connector0/DIO8"=FALSE ("Connector1/DIO39")) -> ()  [unwired: 1 in, 1 out]
        n187 = call "Wait4"("Count(uSec)"=u32 20000) -> ()  [unwired: 1 out]
      }
    }
  }
  n188 = while {
    stop <- FALSE stop-if-true
    n189 = flat-sequence {
      frame #0 {
        n190 = Unbundle By Name("Servo 1 times") -> ("Servo on time"=w423:u32, "Servo off time"=w422:u32)
        n191 = xnode "FPGA I/O Node"("Connector0/DIO9"=TRUE ("Connector1/DIO39")) -> ()  [unwired: 1 in, 1 out]
        n192 = Select(t=w423, s="Servo 1", f=w422) -> (s? t:f=w425:u32)
        n193 = call "Wait6"("Count(uSec)"=w425) -> ()  [unwired: 1 out]
      }
      frame #1 {
        n194 = xnode "FPGA I/O Node"("Connector0/DIO9"=FALSE ("Connector1/DIO39")) -> ()  [unwired: 1 in, 1 out]
        n195 = call "Wait7"("Count(uSec)"=u32 20000) -> ()  [unwired: 1 out]
      }
    }
  }
  n196 = while {
    stop <- FALSE stop-if-true
    n197 = flat-sequence {
      frame #0 {
        n198 = Unbundle By Name("Servo 2 times") -> ("Servo on time"=w432:u32, "Servo off time"=w431:u32)
        n199 = xnode "FPGA I/O Node"("Connector0/DIO10"=TRUE ("Connector1/DIO39")) -> ()  [unwired: 1 in, 1 out]
        n200 = Select(t=w432, s="Servo 2", f=w431) -> (s? t:f=w434:u32)
        n201 = call "Wait8"("Count(uSec)"=w434) -> ()  [unwired: 1 out]
      }
      frame #1 {
        n202 = xnode "FPGA I/O Node"("Connector0/DIO10"=FALSE ("Connector1/DIO39")) -> ()  [unwired: 1 in, 1 out]
        n203 = call "Wait9"("Count(uSec)"=u32 20000) -> ()  [unwired: 1 out]
      }
    }
  }
  n204 = while {
    stop <- FALSE stop-if-true
    n205 = flat-sequence {
      frame #0 {
        n206 = Unbundle By Name("Servo 3 times") -> ("Servo on time"=w441:u32, "Servo off time"=w440:u32)
        n207 = xnode "FPGA I/O Node"("Connector0/DIO11"=TRUE ("Connector1/DIO39")) -> ()  [unwired: 1 in, 1 out]
        n208 = Select(t=w441, s="Servo 3", f=w440) -> (s? t:f=w443:u32)
        n209 = call "Wait10"("Count(uSec)"=w443) -> ()  [unwired: 1 out]
      }
      frame #1 {
        n210 = xnode "FPGA I/O Node"("Connector0/DIO11"=FALSE ("Connector1/DIO39")) -> ()  [unwired: 1 in, 1 out]
        n211 = call "Wait11"("Count(uSec)"=u32 20000) -> ()  [unwired: 1 out]
      }
    }
  }
  n212 = while {
    stop <- FALSE stop-if-true
    n213 = local read "start sequence"() -> (w450:bool)
    n214 = local read "Enum"() -> (w452:enum16{"Pulse", "Fluorescence"})
    n215 = Equal?(x=w452, y=enum16{"Pulse", "Fluorescence"}."Pulse" ("Enum")) -> (x = y?=w451:bool)
    n216 = And(x=w450, y=w451) -> (x .and. y?=w449:bool)
    n217 = case shown="True" w449 {
      frame False {
      }
      frame True {
        n218 = local read "Seq AO bits"() -> (w456:u8)
        n219 = Number To Boolean Array(number=w456) -> (Boolean array=w457:bool[])
        n220 = Array To Cluster(array=w457) -> (cluster=w458:T7)
        n221 = Unbundle(w458) -> ("Boolean array[0]"=w454:bool, "Boolean array[1]"=w455:bool, "Boolean array[2]"=w468:bool)  [unwired: 1 out]
        n222 = Select(t="AO2 on", s=w455, f="AO2 off") -> (s? t:f=w459:i16)
        n223 = Select(t="AO1 on", s=w454, f="AO1 off") -> (s? t:f=w465:i16)
        n224 = Select(t="AO3 on", s=w468, f="AO3 off") -> (s? t:f=w460:i16)
        n225 = xnode "FPGA I/O Node"("Connector0/AO1"=w465, "Connector0/AO2"=w459, "Connector0/AO3"=w460) -> ()  [unwired: 3 in, 3 out]
      }
    }
  }
  n226 = while {
    stop <- FALSE stop-if-true
    n227 = xnode "FPGA I/O Node"("Connector0/AO5"="AO5", "Connector0/AO6"="AO6", "Connector0/AO7"="AO7") -> ()  [unwired: 3 in, 3 out]
  }
  "Slave loop selector" <- u8 0 ("Slave loop selector")
